vi "Insert Redo Command.vi"(8 "error in (no error)":errorcluster, 10 "Redo Command":refnum<class "Undoable Tool.lvclass">, 11 "Stack in":refnum<class "Stack.lvclass">) -> (0 "error out":errorcluster, 1 "Overflow":bool, 2 "Overflow Redo Command":refnum<class "Undoable Tool.lvclass">, 3 "Stack out":refnum<class "Stack.lvclass">)   [LabVIEW 2020, in "Map Model.lvlib" / "Stack.lvclass"]
uses:
  Stack.lvclass
  Tools/Undoable Tool/Undoable Tool.lvclass
  Stack.lvclass/Stack.ctl
panel:
  # "NOTICE -- YOU MUST LEAVE THIS NOTICE IN PLACE.\n\nCopyright (c) 2017, LIANG LIU Shawn.Liu.cn@gmail.com\nAll rights reserved.\n\nRedistribution and use in source and binary forms, with or without modification, are permitted provided that the following conditions are met:\n-Redistributions of source code must retain the above copyright notice, this list of conditions and the following disclaimer.\n-Redistributions in binary form must reproduce the above copyright notice, this list of conditions and the following disclaimer in the documentation and/or other materials provided with the distribution.\n-Neither the name of the eLp nor the names of its contributors may be used to endorse or promote products derived from this software without specific prior written permission.\n\nTHIS SOFTWARE IS PROVIDED BY THE COPYRIGHT HOLDERS AND CONTRIBUTORS \"AS IS\" AND ANY EXPRESS OR IMPLIED WARRANTIES, INCLUDING, BUT NOT LIMITED TO, THE IMPLIED WARRANTIES OF MERCHANTABILITY AND FITNESS FOR A PARTICULAR PURPOSE ARE DISCLAIMED. IN NO EVENT SHALL THE COPYRIGHT HOLDER OR CONTRIBUTORS BE LIABLE FOR ANY DIRECT, INDIRECT, INCIDENTAL, SPECIAL, EXEMPLARY, OR CONSEQUENTIAL DAMAGES (INCLUDING, BUT NOT LIMITED TO, PROCUREMENT OF SUBSTITUTE GOODS OR SERVICES; LOSS OF USE, DATA, OR PROFITS; OR BUSINESS INTERRUPTION) HOWEVER CAUSED AND ON ANY THEORY OF LIABILITY, WHETHER IN CONTRACT, STRICT LIABILITY, OR TORT (INCLUDING NEGLIGENCE OR OTHERWISE) ARISING IN ANY WAY OUT OF THE USE OF THIS SOFTWARE, EVEN IF ADVISED OF THE POSSIBILITY OF SUCH DAMAGE."
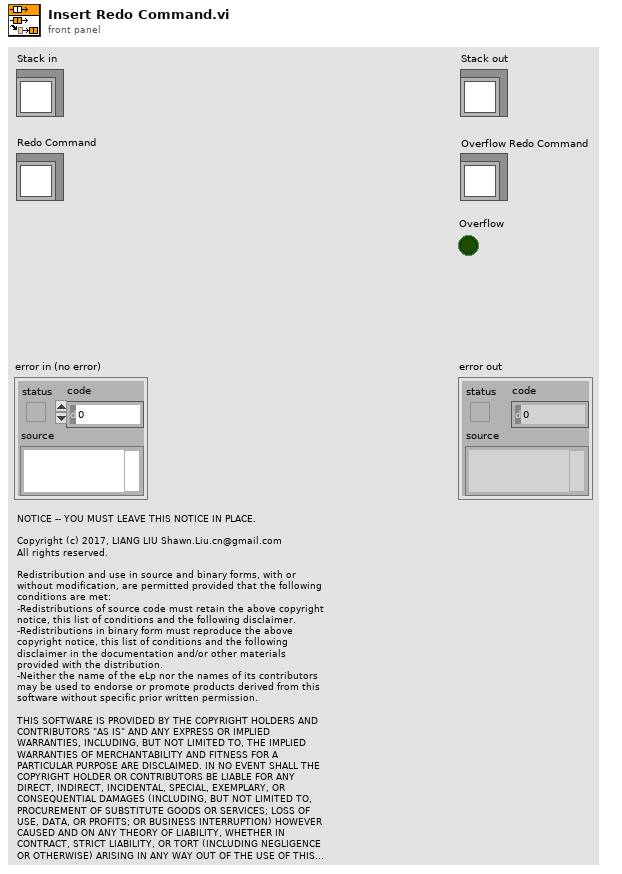
[diagram p1: front panel]
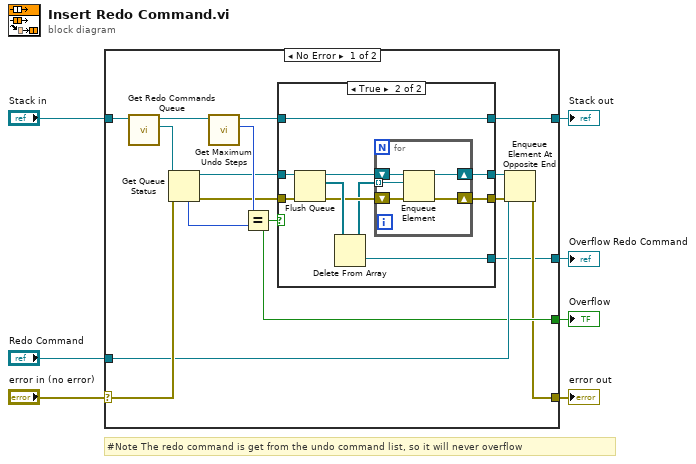
[diagram p0: block diagram]
diagram:
  # "#Note The redo command is get from the undo command list, so it will never overflow"
  n1 = case shown="No Error" "error in (no error)" {
    selector: "error in (no error)" -> [w22 w43]
    tunnel: "Stack in" -> [w23 w42]
    tunnel: [w21 w42] -> w6
    tunnel: "Redo Command" -> [w20 _]
    tunnel: [w19 _] -> w4
    tunnel: [w18 w43] -> w3
    tunnel: [w17 _] -> w5
    frame No Error {
      n2 = call "Get Redo Commands Queue.vi"("Stack in"=w23) -> ("Redo Commands Queue"=w15:refnum<queue>, "Stack out"=w16:refnum<class "Stack.lvclass">)  [unwired: 9 in]
      n3 = Get Queue Status(queue=w15, error in (no error)=w22) -> (queue out=w12:refnum<queue>, error out=w11:errorcluster, # elements in queue=w13:i32)  [unwired: 1 in, 5 out]
      n4 = call "Get Maximum Undo Steps.vi"("Stack in"=w16) -> ("Maximum Undo Steps"=w14:i32, "Stack out"=w10:refnum<class "Stack.lvclass">)  [unwired: 9 in]
      n5 = Equal?(x=w14, y=w13) -> (x = y?=w19:bool)
      n6 = case shown="True" w19 {
        tunnel: w12 -> [w25 w33]
        tunnel: w11 -> [w24 w35]
        tunnel: [_ w34] -> w17
        tunnel: w10 -> [w26 w36]
        tunnel: [w26 w36] -> w21
        tunnel: [w25 w28] -> w9
        tunnel: [w24 w29] -> w8
        frame False {
        }
        frame True {
          n7 = Flush Queue(queue=w33, error in (no error)=w35) -> (queue out=w31:refnum<queue>, remaining elements=w32:refnum<class "Undoable Tool.lvclass">[], error out=w30:errorcluster)
          n8 = Delete From Array(array=w32) -> (deleted portion=w34:refnum<class "Undoable Tool.lvclass">, array with subset deleted=w27:refnum<class "Undoable Tool.lvclass">[])  [unwired: 2 in]
          n9 = for {
            shift-right: [w40] -> w29
            shift-left: w30 -> [w41]
            shift-right: [w38] -> w28
            shift-left: w31 -> [w39]
            tunnel: w27 -> [w37] mode=indexing
            n10 = Enqueue Element(queue=w39, element=w37, error in (no error)=w41) -> (queue out=w38:refnum<queue>, error out=w40:errorcluster)  [unwired: 1 in, 1 out]
          }
        }
      }
      n11 = Enqueue Element At Opposite End(queue=w9, element=w20, error in (no error)=w8) -> (error out=w18:errorcluster)  [unwired: 1 in, 2 out]
    }
    frame Error {
    }
  }
  "error out" <- w3
  "Stack out" <- w6
  "Overflow Redo Command" <- w5
  "Overflow" <- w4
